vi "dvp Vi Set Strobe Output Type.vi"(10 "StrobeOutputType":u32(ring) items=["STROBE_OUT_OFF", "STROBE_OUT_LOW", "STROBE_OUT_HIGH"], 11 "handle":u32) -> (3 "function return":u32(ring))   [LabVIEW 2018, in "LabViewDVPCamera.lvlib"]
doc: "LabviewDvp2Api dvpStatus dvpViSetStrobeOutputType(dvpHandle handle, dvpStrobeOutputType StrobeOutputType);"
uses:
  LabViewDVPCamera.lvlib
  LabViewDVPCamera/LabViewDVPCamera.dll
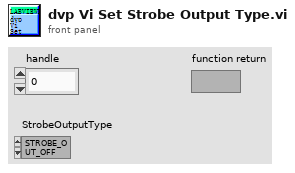
[diagram p1: front panel]
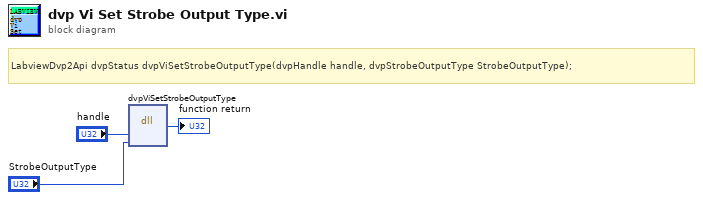
[diagram p0: block diagram]
diagram:
  # "LabviewDvp2Api dvpStatus dvpViSetStrobeOutputType(dvpHandle handle, dvpStrobeOutputType StrobeOutputType);"
  n1 = dll-call lib="C:/Program Files (x86)/DVP2 Labview cn 64/Sample/LabViewDVPCamera/LabViewDVPCamera.*" fn="dvpViSetStrobeOutputType"("handle"="handle", "StrobeOutputType"="StrobeOutputType") -> (→"function return":u32)  [unwired: 5 in, 2 out]
